vi "array index series feb 11 2016.vi"() -> ()   [LabVIEW 2015]
panel:
  in  "Array":cluster{"Numeric":dbl, "Numeric 2":dbl}[](array[cluster])
  out "Boolean 2":bool
  out "Array 2":dbl[][](array[numeric])
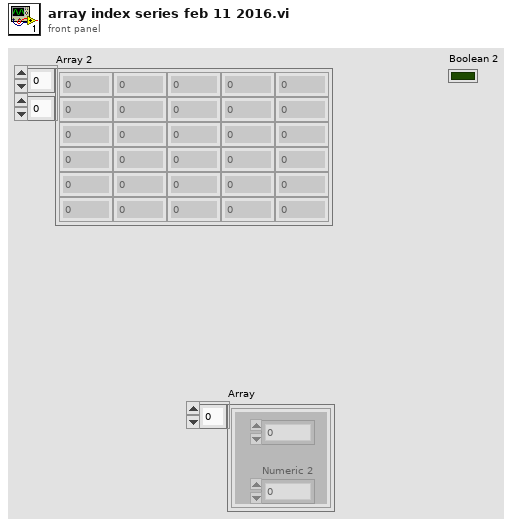
[diagram p1: front panel]
types:
  T1 = cluster{"Array 2[0]":dbl, "Array 2[1]":dbl, "Array 2[2]":dbl, "Array 2[3]":dbl, "Array 2[4]":dbl, "Array 2[5]":dbl, "Array 2[6]":dbl, "Array 2[7]":dbl, "Array 2[8]":dbl}
  T2 = cluster{cluster{"Array 2[0]":dbl, "Array 2[1]":dbl}}
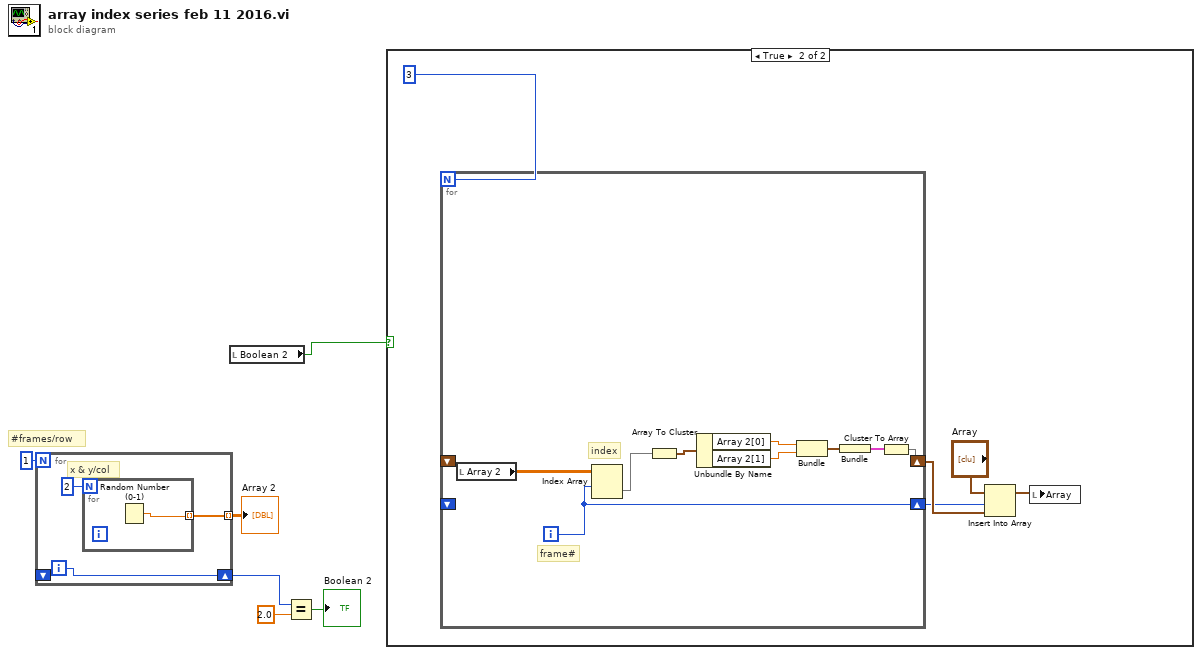
[diagram p0: block diagram]
diagram:
  # "#frames/row"
  n1 = for {
    N: 1 -> [_]
    tunnel: [w9] -> w6 mode=indexing
    shift-right: [w7] -> w1
    shift-left: _ -> [_]
    i -> [w7]
    # "x & y/col"
    n2 = for {
      N: 2 -> [_]
      tunnel: [w10] -> w9 mode=indexing
      n3 = Random Number (0-1)() -> (number: 0 to 1=w10:dbl)
    }
  }
  "Array 2" <- w6
  n4 = local read "Boolean 2"() -> (w4:bool)
  n5 = Equal?(x=w1, y=2.0) -> (x = y?=→"Boolean 2":bool)
  n6 = case shown="True" w4 {
    frame False {
    }
    frame True {
      n7 = for {
        N: 3 -> [_]
        shift-right: [w17] -> w14
        shift-left: _ -> [_]
        shift-right: [w16] -> w11
        shift-left: _ -> [_]
        i -> [w16]
        # "frame#"
        # "index"
        n8 = local read "Array 2"() -> (w24:dbl[][])
        n9 = Index Array(array=w24, index (row)=w16) -> (element=w23:dbl[])  [unwired: 1 in]
        n10 = Array To Cluster(array=w23) -> (cluster=w22:T1)
        n11 = Unbundle By Name(w22) -> ("Array 2[0]"=w21:dbl, "Array 2[1]"=w20:dbl)
        n12 = Bundle("Array 2[0]"=w21, "Array 2[1]"=w20) -> (w19:cluster{"Array 2[0]":dbl, "Array 2[1]":dbl})  [unwired: 1 in]
        n13 = Bundle(w19) -> (w18:T2)  [unwired: 1 in]
        n14 = Cluster To Array(cluster=w18) -> (array=w17:cluster{"Array 2[0]":dbl, "Array 2[1]":dbl}[])
      }
      n15 = Insert Into Array(array="Array", index=w11, new element=w14) -> (w12:cluster{"Numeric":dbl, "Numeric 2":dbl}[])
      n16 = local write "Array"(w12) -> ()
    }
  }
